vi "FGVChannels.vi"(6 "Units/Cal/Offset In":T3, 7 "Enum":T4, 8 "error in":errorcluster, 9 "channelsNamesIn":string[](array[string]), 10 "SavingChoiceIn":T1, 11 "XYZ Units/Cal/Offset In":T3) -> (0 "error out":errorcluster, 1 "channelsNamesOut":string[](array[string]), 2 "SavingChoiceOut":T2, 3 "XYZ Units/Cal/Offset Out":T3, 4 "Units/Cal/Offset Out":T3)   [LabVIEW 2016]
uses:
  controls/Enum.ctl
  <vilib>/rvi/interface/nirviReadWriteControl/nirviReadWriteControl.xnode
  controls/FPGAVIreferenceTypeDef.ctl
  FPGA Bitfiles/lbniAFMControlle_flexRio_controllerFPGA.lvbitx
  NiFpgaLv.dll
  <vilib>/Utility/error.llb/Error Cluster From Error Code.vi
  <vilib>/rvi/errors/niLvFpgaAdjustHostInterfaceError.vi
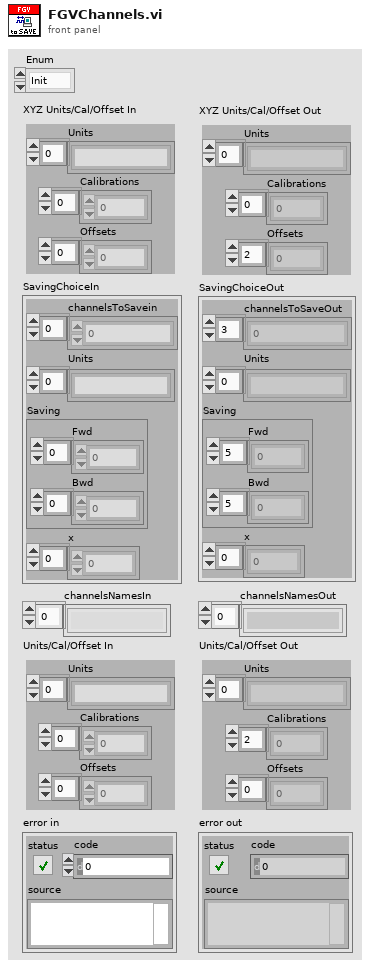
[diagram p1: front panel]
types:
  T1 = cluster{"channelsToSavein":u8[], "Units":string[], "Saving":cluster{"Fwd":i32[], "Bwd":i32[]}, "x":i32[]}
  T2 = cluster{"channelsToSaveOut":u8[], "Units":string[], "Saving":cluster{"Fwd":i32[], "Bwd":i32[]}, "x":i32[]}
  T3 = cluster{"Units":string[], "Offsets":dbl[], "Calibrations":dbl[]}
  T4 = typedef "Enum.ctl" = enum16{"Init", "Read", "Write"}
  T5 = typedef "FPGAVIreferenceTypeDef.ctl" = refnum<k20>
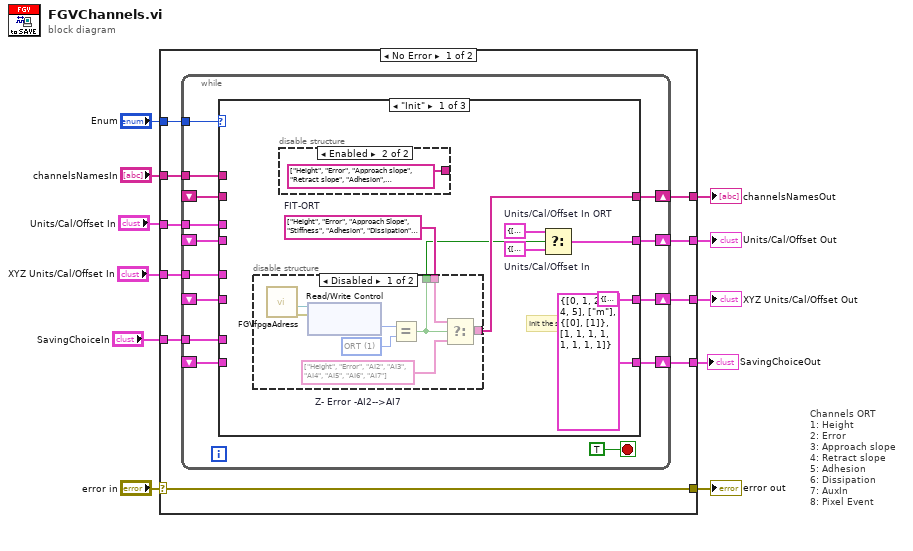
[diagram p0: block diagram]
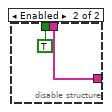
[diagram p2: hidden frame]
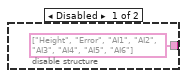
[diagram p3: hidden frame]
diagram:
  # "Channels ORT\n1: Height\n2: Error\n3: Approach slope\n4: Retract slope\n5: Adhesion\n6: Dissipation\n7: AuxIn\n8: Pixel Event"
  n1 = case shown="No Error" "error in" {
    selector: "error in" -> [w20 w68]
    tunnel: "Enum" -> [w21 _]
    tunnel: [w20 w68] -> w10
    tunnel: [w18 w67] -> w7
    tunnel: "channelsNamesIn" -> [w19 w67]
    tunnel: "Units/Cal/Offset In" -> [w17 w66]
    tunnel: [w16 w66] -> w5
    tunnel: "XYZ Units/Cal/Offset In" -> [w15 w65]
    tunnel: [w14 w65] -> w3
    tunnel: "SavingChoiceIn" -> [w13 w64]
    tunnel: [w12 w64] -> w2
    frame No Error {
      n2 = while {
        tunnel: w21 -> [w34]
        tunnel: w19 -> [w33]
        shift-right: [w32] -> w18
        shift-left: _ -> [w31]
        tunnel: w17 -> [w30]
        shift-right: [w29] -> w16
        shift-left: _ -> [w28]
        tunnel: w15 -> [w27]
        shift-right: [w26] -> w14
        shift-left: _ -> [w25]
        tunnel: w13 -> [w24]
        shift-right: [w23] -> w12
        shift-left: _ -> [w22]
        stop <- TRUE stop-if-true
        n3 = case shown="\"Init\"" w34 {
          tunnel: w33 -> [_ _ w63]
          tunnel: [w42 w59 w63] -> w32
          tunnel: w31 -> [_ w59 _]
          tunnel: w30 -> [_ _ w62]
          tunnel: [w38 w58 w62] -> w29
          tunnel: w28 -> [_ w58 _]
          tunnel: w27 -> [_ _ w61]
          tunnel: [T3 {"Units"=["m", "m", "m"], "Offsets"=[0.0, 0.0, 0.0], "Calibrations"=[1.0, 1.0, 1.0]} ("XYZ Units/Cal/Offset In") w57 w61] -> w26
          tunnel: w25 -> [_ w57 _]
          tunnel: w24 -> [_ _ w60]
          tunnel: [T2 {"channelsToSaveOut"=[0, 1, 2, 3, 4, 5], "Units"=["m"], "Saving"={"Fwd"=[0], "Bwd"=[1]}, "x"=[1, 1, 1, 1, 1, 1, 1, 1]} ("SavingChoiceOut") w56 w60] -> w23
          tunnel: w22 -> [_ w56 _]
          frame "Init" {
            w40 = T3 {"Units"=["V", "V", "V", "V", "V", "V", "V", "V"], "Offsets"=[0.0, 0.0, 0.0, 0.0, 0.0, 0.0, 0.0, 0.0], "Calibrations"=[1.0, 1.0, 1.0, 1.0, 1.0, 1.0, 1.0, 1.0]}  # Units/Cal/Offset In ORT
            w41 = T3 {"Units"=["V", "V", "V", "V", "V", "V", "V", "V"], "Offsets"=[0.0, 0.0, 0.0, 0.0, 0.0, 0.0, 0.0, 0.0], "Calibrations"=[1.0, 1.0, 1.0, 1.0, 1.0, 1.0, 1.0, 1.0]}  # Units/Cal/Offset In
            w43 = string[] ["Height", "Error", "Approach Slope", "Stiffness", "Adhesion", "Dissipation", "Aux In (AI1)", "Pixel Event"]  # FIT-ORT
            # "Init the saving\nChannels"
            n4 = disable-structure shown="Disabled" {
              disable-tunnel: w43 -> [w46 w53]
              disable-tunnel: [w45 w53] -> w42
              disable-tunnel: [w44 TRUE] -> w39
              frame Disabled {
                w47 = string[] ["Height", "Error", "AI2", "AI3", "AI4", "AI5", "AI6", "AI7"]  # Z- Error -AI2-->AI7
                w48 = u8 1 items=["Contact Mode", "ORT", "Aux"] ("fb.i.source")
                n5 = call "FGVfpgaAdress.vi"() -> ("error out"=w51:errorcluster, "FPGA VI Reference Out"=w50:T5)  [unwired: 6 in, 4 out]
                n6 = xnode "Read/Write Control"("FPGA VI Reference In"=w50, "error in"=w51) -> ("fb.i.source"=w49:u8)  [unwired: 2 out]
                n7 = Equal?(x=w49, y=w48) -> (x = y?=w44:bool)
                n8 = Select(t=w46, s=w44, f=w47) -> (s? t:f=w45:string[])
              }
              frame Enabled {
              }
            }
            n9 = disable-structure shown="Enabled" {
              disable-tunnel: [string[] ["Height", "Error", "AI1", "AI2", "AI3", "AI4", "AI5", "AI6"] ("channelsNamesIn") string[] ["Height", "Error", "Approach slope", "Retract slope", "Adhesion", "Dissipation", "AuxIn", "Aux", "AI0", "AI1", "AI2", "AI3", "AI4", "AI5", "AI6", "AI7"] ("channelsNamesIn")] -> _
              frame Disabled {
              }
              frame Enabled {
              }
            }
            n10 = Select(t=w40, s=w39, f=w41) -> (s? t:f=w38:T3)
          }
          frame "Read", Default {
          }
          frame "Write" {
          }
        }
      }
    }
    frame Error {
    }
  }
  "error out" <- w10
  "channelsNamesOut" <- w7
  "Units/Cal/Offset Out" <- w5
  "XYZ Units/Cal/Offset Out" <- w3
  "SavingChoiceOut" <- w2
